vi "RT Pin Test.vi"() -> ()   [LabVIEW 2015]
uses:
  <vilib>/rvi/interface/nirviOpenFPGA/nirviOpenFPGA.xnode
  FPGA Bitfiles/Puppy_FPGATarget9607_FPGAPinTest_9O48HGQC5kI.lvbitx
  <vilib>/FPGAPlugInAG/sbRIO-9607/niLvFpga_Open_sbRIO-9607.vi
  <vilib>/rvi/interface/nirviReadWriteControl/nirviReadWriteControl.xnode
  <vilib>/rvi/interface/nirviMethod/nirviMethod.xnode
  <vilib>/FPGAPlugInAG/sbRIO-9607/niLvFpga_Reset_sbRIO-9607.vi
  <vilib>/FPGAPlugInAG/sbRIO-9607/niLvFpga_Run_sbRIO-9607.vi
  NiFpgaLv.dll
  <vilib>/Utility/error.llb/Error Cluster From Error Code.vi
  <vilib>/rvi/errors/niLvFpgaAdjustHostInterfaceError.vi
  <vilib>/FPGAPlugInAG/sbRIO-9607/niLvFpga_Abort_sbRIO-9607.vi
  <vilib>/rvi/interface/nirviCloseFPGA/nirviCloseFPGA.xnode
  <vilib>/FPGAPlugInAG/sbRIO-9607/niLvFpga_Close_sbRIO-9607.vi
panel:
  out "Digtal IO/DIO54":bool
  in  "Digtal IO/DIO55":bool
  in  "Stop Button":bool
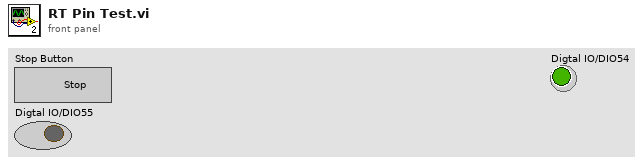
[diagram p1: front panel]
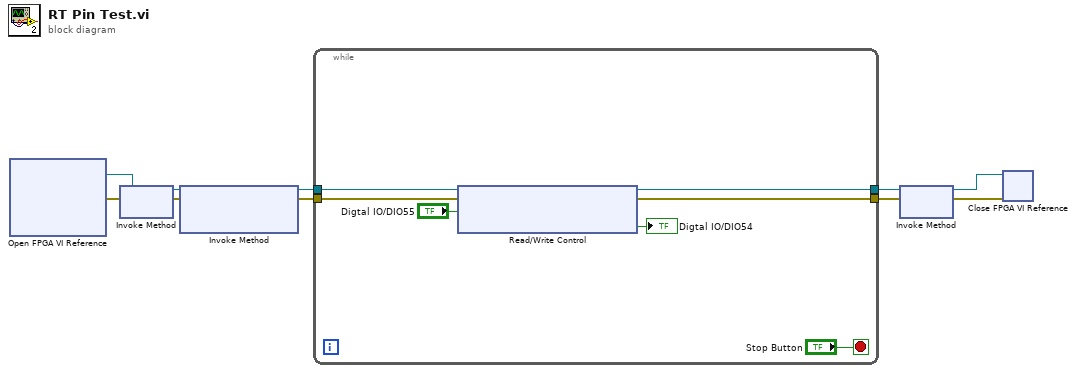
[diagram p0: block diagram]
diagram:
  n1 = xnode "Open FPGA VI Reference"() -> ("FPGA VI Reference Out"=w10:refnum<k20>, "error out"=w9:errorcluster)  [unwired: 2 in]
  n2 = xnode "Invoke Method"("FPGA VI Reference In"=w10, "error in"=w9) -> ("FPGA VI Reference Out"=w8:refnum<k20>, "error out"=w7:errorcluster)
  n3 = xnode "Invoke Method"("FPGA VI Reference In"=w8, "error in"=w7) -> ("FPGA VI Reference Out"=w6:refnum<k20>, "error out"=w5:errorcluster)  [unwired: 1 in]
  n4 = while {
    tunnel: w6 -> [w16]
    tunnel: w5 -> [w15]
    tunnel: [w12] -> w4
    tunnel: [w11] -> w3
    stop <- "Stop Button" stop-if-true
    n5 = xnode "Read/Write Control"("FPGA VI Reference In"=w16, "error in"=w15, "Digtal IO/DIO55"="Digtal IO/DIO55") -> ("FPGA VI Reference Out"=w12:refnum<k20>, "error out"=w11:errorcluster, "Digtal IO/DIO54"=→"Digtal IO/DIO54":bool)
  }
  n6 = xnode "Invoke Method"("FPGA VI Reference In"=w4, "error in"=w3) -> ("FPGA VI Reference Out"=w1:refnum<k20>, "error out"=w2:errorcluster)
  n7 = xnode "Close FPGA VI Reference"("FPGA VI Reference In"=w1, "error in"=w2) -> ()  [unwired: 1 out]
